vi "Fibonacci array.vi"() -> ()   [LabVIEW 2013]
panel:
  out "数组 3":i32[](array[numeric])
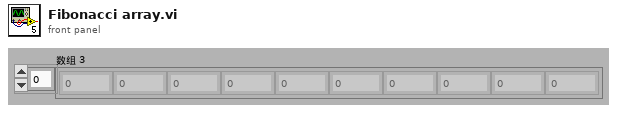
[diagram p1: front panel]
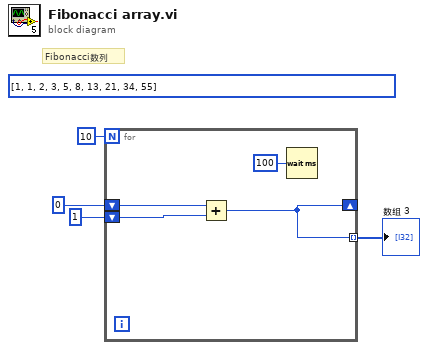
[diagram p0: block diagram]
diagram:
  (unwired) i32[] [1, 1, 2, 3, 5, 8, 13, 21, 34, 55] ("数组 3")
  # "Fibonacci数列"
  n1 = for {
    N: 10 -> [_]
    shift-right: [w6] -> _
    shift-left: 0 -> [w8]
    shift-left: 1 -> [w7]
    tunnel: [w6] -> w1 mode=indexing
    n2 = Add(x=w8, y=w7) -> (x+y=w6:i32)
    n3 = Wait (ms)(milliseconds to wait=u32 100 ("等待时间（毫秒）")) -> ()  [unwired: 1 out]
  }
  "数组 3" <- w1
